vi "parse_MultiArrayDimension.vi"(4 "error in":errorcluster, 7 "msg in":string) -> (0 "error out":errorcluster, 2 "Array":T1, 3 "msg out":string)   [LabVIEW 2015]
doc: "Parses a message into a multi array dimension"
uses:
  subs/parse_string_scalar.vi
  subs/parse_u32_scalar.vi
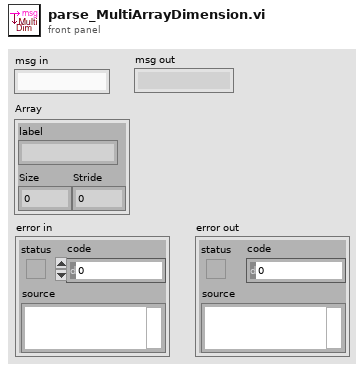
[diagram p1: front panel]
types:
  T1 = cluster{"label":string, "Size":u32, "Stride":u32}
  T2 = cluster{"Label":string, "Size":u32, "Stride":u32}
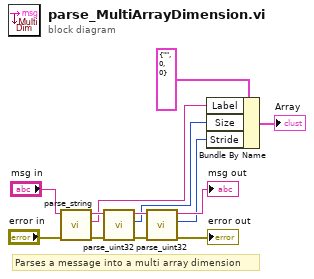
[diagram p0: block diagram]
diagram:
  # "Parses a message into a multi array dimension"
  n1 = call-poly "parse_string.vi"("error in"="error in", "msg in"="msg in") -> ("error out"=w13:errorcluster, "string"=w5:string, "msg out"=w12:string)  [unwired: 3 in]
  n2 = call-poly "parse_uint32.vi"("error in"=w13, "msg in"=w12) -> ("error out"=w11:errorcluster, "number"=w4:u32, "msg out"=w8:string)  [unwired: 3 in]
  n3 = call-poly "parse_uint32.vi"("error in"=w11, "msg in"=w8) -> ("error out"=→"error out":errorcluster, "number"=w3:u32, "msg out"=→"msg out":string)  [unwired: 3 in]
  n4 = Bundle By Name(cluster=T2 {"Label"="", "Size"=0, "Stride"=0} ("input cluster"), "Label"=w5, "Size"=w4, "Stride"=w3) -> (→"Array":T2)
